vi "WaitTimes.vi"(6 "WaitTimes":u32, 8 "error in (no error)":errorcluster caption="ErrorIn") -> (0 "error out":errorcluster caption="ErrorOut")   [LabVIEW 2013]
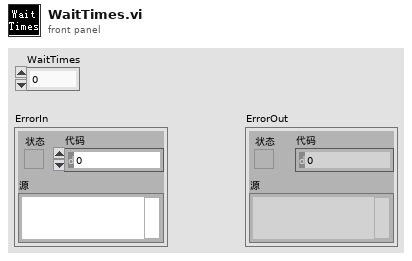
[diagram p1: front panel]
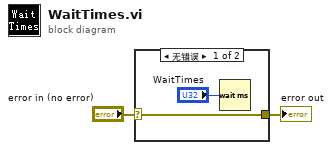
[diagram p0: block diagram]
diagram:
  n1 = case shown="无错误" "error in (no error)" {
    selector: "error in (no error)" -> [w3 w5]
    tunnel: [w3 w5] -> w1
    frame No Error {
      n2 = Wait (ms)(milliseconds to wait="WaitTimes") -> ()  [unwired: 1 out]
    }
    frame Error {
    }
  }
  "error out" <- w1
